vi "Destroy.vi"(0 "reference in":refnum<class "G#SubClass2.lvclass">, 5 "error in (no error)":errorcluster) -> (14 "reference out":refnum<class "G#SubClass2.lvclass">, 19 "error out":errorcluster)   [LabVIEW 2020, in "G#SubClass2.lvclass"]
doc: "Destructor."
uses:
  G#SubClass2.lvclass
  C:/Program Files (x86)/National Instruments/LabVIEW 2020/vi.lib/addons/_AddQ/G#Object/G#Object.lvclass
  G#BaseClass2_class/G#BaseClass2.lvclass
  <vilib>/addons/_AddQ/G#Object/G#Object.lvclass
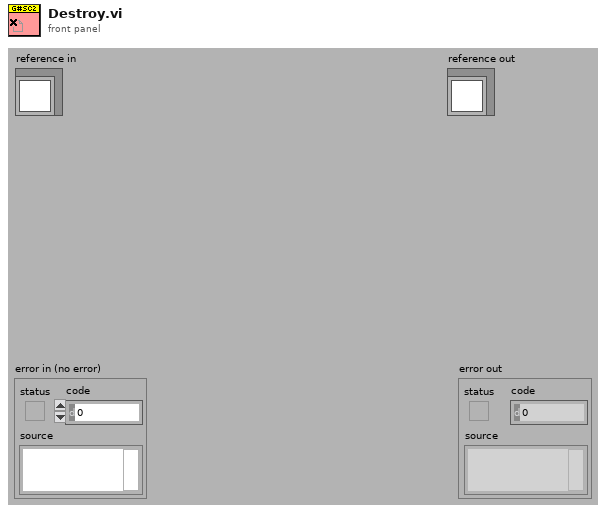
[diagram p1: front panel]
types:
  T1 = typedef "G#SubClass2.lvclass/ObjectAttributes.ctl" = cluster{"Base class":T2, "SubAttribute":dbl}
  T2 = typedef "G#BaseClass2.lvclass/ObjectAttributes.ctl" = cluster{"Numeric":dbl, "Array":dbl[]}
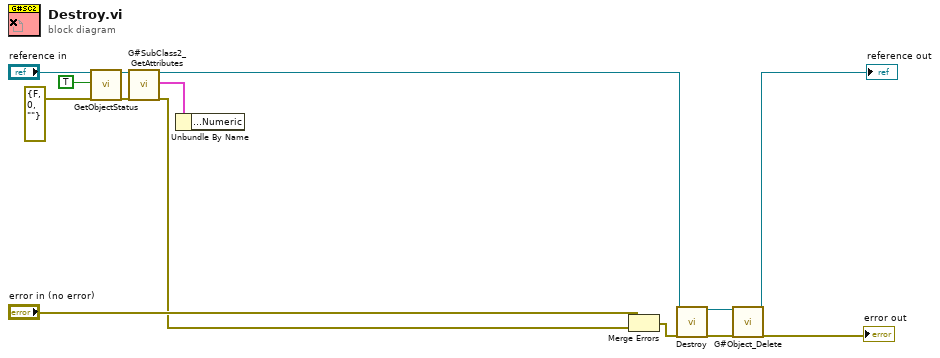
[diagram p0: block diagram]
diagram:
  n1 = call-dynamic "GetObjectStatus.vi"("reference in"="reference in", "simple info (F)"=TRUE ("simple info"), "error in (no error)"=errorcluster {"status"=FALSE, "code"=0, "source"=""}) -> ("reference out"=w4:refnum<class "G#SubClass2.lvclass">, "error out"=w5:errorcluster)  [unwired: 5 in, 10 out]
  n2 = call "G#SubClass2_GetAttributes.vi"("reference in"=w4, "error in (no error)"=w5) -> ("reference out"=w11:refnum<class "G#SubClass2.lvclass">, "attributes"=w6:T1, "error out"=w7:errorcluster)  [unwired: 14 in, 1 out]
  n3 = Unbundle By Name(w6) -> ()  [unwired: 1 out]
  n4 = Merge Errors("error in (no error)", w7) -> (w12:errorcluster)
  n5 = call-parent "Destroy.vi"("reference in"=w11, "error in (no error)"=w12) -> ("reference out"=w9:refnum<class "G#SubClass2.lvclass">, "error out"=w10:errorcluster)  [unwired: 16 in]
  n6 = call <vilib>:"G#Object_Delete.vi"("reference in"=w9, "error in (no error)"=w10) -> ("reference out"=→"reference out":refnum<class "G#SubClass2.lvclass">, "error out"=→"error out":errorcluster)  [unwired: 16 in]
